vi "Config Write Channels.vi"(8 "error in (no error)":errorcluster, 10 "Channels In":T2[](array[typedef]) {"Mapping"."VS Reference" format="%.0x"}, 11 "Refnum in":T1) -> (0 "error out":errorcluster, 3 "Refnum out":T1)   [LabVIEW 2021, in "Modbus Master System Explorer.lvlib"]
uses:
  Modbus Master System Explorer.lvlib
  <vilib>/Utility/config.llb/Config Data RefNum.ctl
  Shared/Controls/Data Model/Channel.ctl
  Modbus Type.ctl
  <vilib>/NI VeriStand/Custom Device API/Custom Device Channel Type.ctl
  Shared/Controls/Data Model/Mapping.ctl
  Shared/Controls/Data Model/DataType.ctl
  <vilib>/NI VeriStand/Custom Device API/Custom Device Item Ref.ctl
  <vilib>/Utility/config.llb/Write Key (String).vi
  <vilib>/Utility/config.llb/Write Key (U32).vi
  <vilib>/Utility/config.llb/NI_LVConfig.lvlib
  <vilib>/NI VeriStand/Custom Device API/Custom Device API.lvlib
  Shared/Modbus Master Shared.lvlib
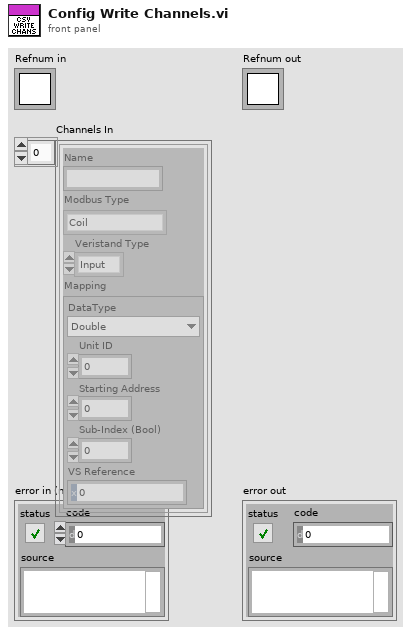
[diagram p1: front panel]
types:
  T1 = typedef "NI_LVConfig.lvlib/Config Data RefNum.ctl" = refnum<k1>
  T2 = typedef "Modbus Master Shared.lvlib/Channel.ctl" = cluster{"Name":string, "Modbus Type":T3, "Veristand Type":T4, "Mapping":T5}
  T3 = typedef "Modbus Master Shared.lvlib/Modbus Type.ctl" = enum16{"Coil", "Discrete Input", "Holding Register", "Input Register"}
  T4 = typedef "Custom Device API.lvlib/Custom Device Channel Type.ctl" = enum16{"Input", "Output"}
  T5 = typedef "Modbus Master Shared.lvlib/Mapping.ctl" = cluster{"DataType":T6, "Unit ID":u8, "Starting Address":u16, "Sub-Index (Bool)":u16, "VS Reference":T7}
  T6 = typedef "Modbus Master Shared.lvlib/DataType.ctl" = enum16{"Double", "Single", "I64", "I32", "I16", "I8", "U64", "U32", "U16", "U8", "Boolean"}
  T7 = typedef "Custom Device API.lvlib/Custom Device Item Ref.ctl" = u64
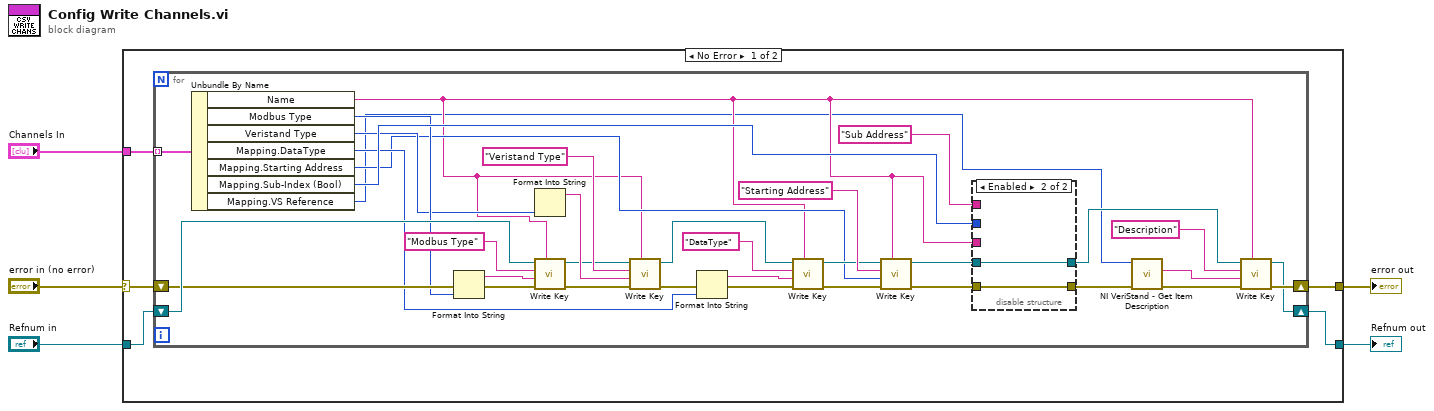
[diagram p0: block diagram]
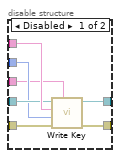
[diagram p2: hidden frame]
diagram:
  n1 = case shown="No Error" "error in (no error)" {
    selector: "error in (no error)" -> [w10 w55]
    tunnel: "Refnum in" -> [w9 w56]
    tunnel: "Channels In" -> [w8 _]
    tunnel: [w7 w55] -> w2
    tunnel: [w6 w56] -> w1
    frame No Error {
      n2 = for {
        shift-right: [w19] -> w7
        shift-left: w10 -> [w33]
        tunnel: w8 -> [w45] mode=indexing
        shift-right: [w17] -> w6
        shift-left: w9 -> [w36]
        n3 = Unbundle By Name(w45) -> ("Name"=w16:string, "Modbus Type"=w32:T3, "Veristand Type"=w30:T4, "Mapping.DataType"=w26:T6, "Mapping.Starting Address"=w20:u16, "Mapping.Sub-Index (Bool)"=w39:u16, "Mapping.VS Reference"=w12:T7)
        n4 = Format Into String(error in=w33, w32) -> (resulting string=w35:string, error out=w34:errorcluster)  [unwired: 2 in]
        n5 = Format Into String(w30) -> (resulting string=w29:string)  [unwired: 3 in, 1 out]
        n6 = call-poly <vilib>:"Write Key.vi"("section"=w16, "error in (no error)"=w34, "value"=w35, "key"="Modbus Type", "refnum"=w36) -> ("error out"=w28:errorcluster, "refnum out"=w27:T1)  [unwired: 4 in, 1 out]
        n7 = call-poly <vilib>:"Write Key.vi"("section"=w16, "error in (no error)"=w28, "value"=w29, "key"="Veristand Type", "refnum"=w27) -> ("error out"=w23:errorcluster, "refnum out"=w25:T1)  [unwired: 4 in, 1 out]
        n8 = Format Into String(error in=w23, w26) -> (resulting string=w37:string, error out=w22:errorcluster)  [unwired: 2 in]
        n9 = call-poly <vilib>:"Write Key.vi"("section"=w16, "error in (no error)"=w22, "value"=w37, "key"="DataType", "refnum"=w25) -> ("error out"=w21:errorcluster, "refnum out"=w24:T1)  [unwired: 4 in, 1 out]
        n10 = call-poly <vilib>:"Write Key.vi"("section"=w16, "error in (no error)"=w21, "value"=w20, "key"="Starting Address", "refnum"=w24) -> ("error out"=w41:errorcluster, "refnum out"=w40:T1)  [unwired: 4 in, 1 out]
        n11 = disable-structure shown="Enabled" {
          disable-tunnel: "Sub Address" ("key") -> [w52 _]
          disable-tunnel: w41 -> [w51 w53]
          disable-tunnel: w40 -> [w50 w54]
          disable-tunnel: w39 -> [w49 _]
          disable-tunnel: [w48 w53] -> w14
          disable-tunnel: [w47 w54] -> w18
          disable-tunnel: w16 -> [w46 _]
          frame Disabled {
            n12 = call-poly <vilib>:"Write Key.vi"("section"=w46, "error in (no error)"=w51, "value"=w49, "key"=w52, "refnum"=w50) -> ("error out"=w48:errorcluster, "refnum out"=w47:T1)  [unwired: 4 in, 1 out]
          }
          frame Enabled {
          }
        }
        n13 = call <vilib>:"NI VeriStand - Get Item Description.vi"("error in (no error)"=w14, "Item Ref in"=w12) -> ("error out"=w13:errorcluster, "Description"=w11:string)  [unwired: 6 in, 2 out]
        n14 = call-poly <vilib>:"Write Key.vi"("section"=w16, "error in (no error)"=w13, "value"=w11, "key"="Description", "refnum"=w18) -> ("error out"=w19:errorcluster, "refnum out"=w17:T1)  [unwired: 4 in, 1 out]
      }
    }
    frame Error {
    }
  }
  "error out" <- w2
  "Refnum out" <- w1
